vi "Set Setpoint Limits--Accessor.vi"(8 "error in (no error)":errorcluster, 10 "Limits":T1, 11 "Watlow F4T in":refnum<class "Watlow F4T.lvclass">) -> (0 "error out":errorcluster, 3 "Watlow F4T out":refnum<class "Watlow F4T.lvclass">)   [LabVIEW 2024, in "Watlow F4T.lvclass"]
uses:
  Watlow F4T.lvclass
  Process Controller/Controls/Limits--Cluster.ctl
  Watlow F4T.lvclass/Watlow F4T.ctl
  Process Controller/_Thermal Process Controller.lvclass
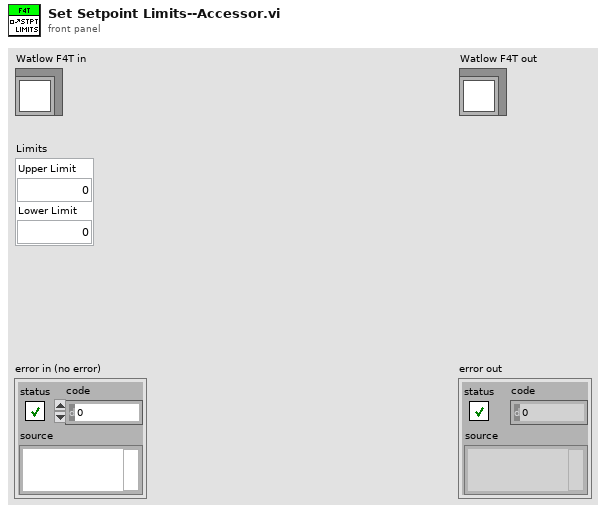
[diagram p1: front panel]
types:
  T1 = typedef "_Thermal Process Controller.lvclass/Limits--Cluster.ctl" = cluster{"Upper Limit":dbl, "Lower Limit":dbl}
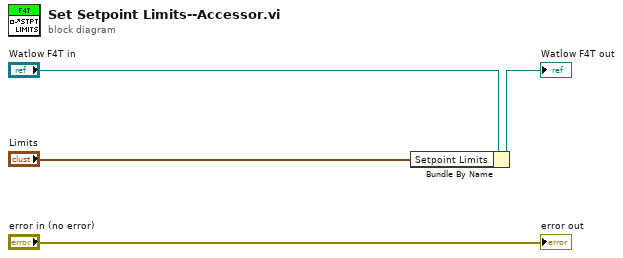
[diagram p0: block diagram]
diagram:
  n1 = Bundle By Name(cluster="Watlow F4T in", "Setpoint Limits"="Limits") -> (→"Watlow F4T out":refnum<class "Watlow F4T.lvclass">)
  "error out" <- "error in (no error)"
